vi "DAQmx Create CI Channel (sub).vi"(0 "task in":refnum<k21>, 1 "virtual channel name":string, 5 "physical channel name":tag, 7 "measurement type":i32(ring)=10125 items=["count events"=10125, "frequency"=10179, "period"=10256, "pulse width"=10359, "semi period"=10289, "pulse frequency"=15864, "pulse time"=15865, "pulse ticks"=15866, "two edge separation"=10267, "angular encoder"=10360, "linear encoder"=10361, "gps timestamp"=10362], 11 "error in":errorcluster, 13 "custom scale":tag) -> (4 "task out":refnum<k21>, 6 "channel names":string, 15 "error out":errorcluster)   [LabVIEW 2011]
uses:
  nilvaiu.dll
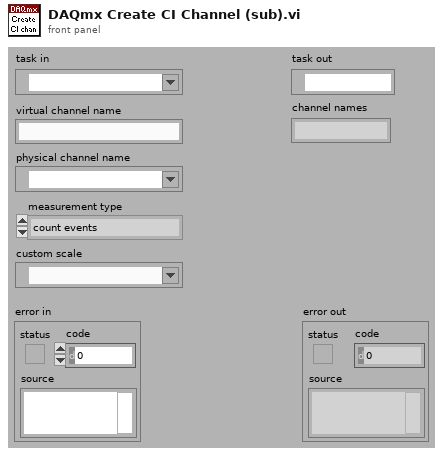
[diagram p1: front panel]
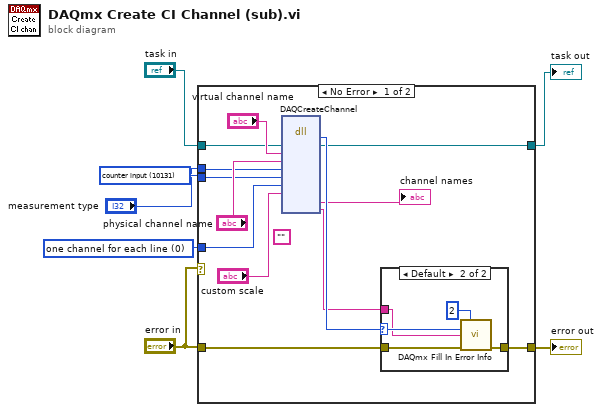
[diagram p0: block diagram]
diagram:
  w3 = 0 items=["one channel for each line", "one channel for all lines"] ("line grouping")
  w4 = 10131 items=["analog input"=10100, "analog output"=10102, "digital input"=10151, "digital output"=10153, "counter input"=10131, "counter output"=10132] ("channel type")
  n1 = case shown="No Error" "error in" {
    tunnel: [w16 w28] -> w7
    tunnel: "error in" -> [w18 w28]
    tunnel: "task in" -> [w8 w27]
    tunnel: "measurement type" -> [w15 _]
    tunnel: w4 -> [w14 _]
    tunnel: w3 -> [w10 _]
    tunnel: [w9 w27] -> w1
    frame No Error {
      (unwired) ""
      n2 = dll-call lib="nilvaiu.*" fn="DAQCreateChannel"("task in"=w8, "virtual chnanel name"="virtual channel name", "physical channel name"="physical channel name", "measurement type"=w15, "channel type"=w14, "line grouping"=w10, "customScale"="custom scale") -> (w17:i32, "task in"=w9:refnum<k21>, "channel names"=→"channel names":string, "extendedErrorIndo"=w11:string)  [unwired: 9 in, 4 out]
      n3 = case shown="Default" w17 {
        selector: w17 -> [_ w24]
        tunnel: w18 -> [w21 w26]
        tunnel: [w21 w25] -> w16
        tunnel: w11 -> [_ w23]
        frame 0 {
        }
        frame Default {
          n4 = call "DAQmx Fill In Error Info.vi"("depth"=2, "status code"=w24, "extended error info"=w23, "error in"=w26) -> ("error out"=w25:errorcluster)  [unwired: 1 in, 10 out]
        }
      }
    }
    frame Error {
    }
  }
  "error out" <- w7
  "task out" <- w1
